vi "VS-Scale Time Axis.vi"(0 "Graph Ref":refnum<vi>, 7 "Running?":bool, 9 "Plot what":T1={"Mode"=enum."all time", "hours"=0.1} {"hours" min=0.1 max=24.0 step=0.5}, 11 "error in (no error)":errorcluster) -> (15 "error out":errorcluster)   [LabVIEW 2020]
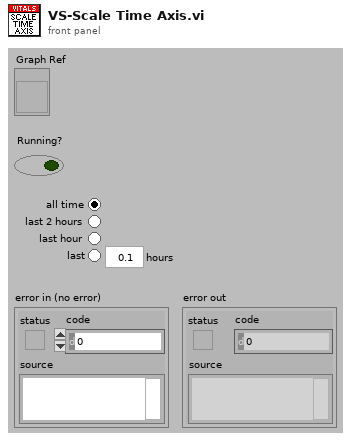
[diagram p1: front panel]
types:
  T1 = cluster{"Mode":enum32{"all time", "last 2 hours", "last hour", "last"}, "hours":dbl}
  T2 = enum32{"all time", "last 2 hours", "last hour", "last"}
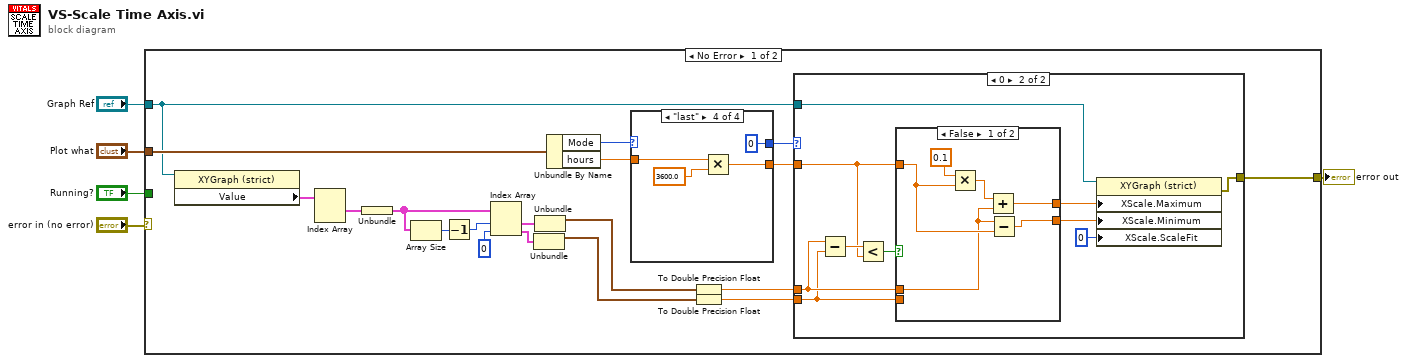
[diagram p0: block diagram]
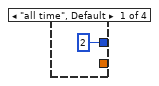
[diagram p2: hidden frame]
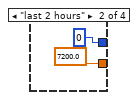
[diagram p3: hidden frame]
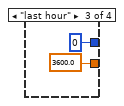
[diagram p4: hidden frame]
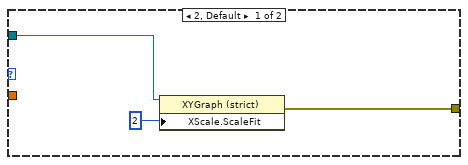
[diagram p5: hidden frame]
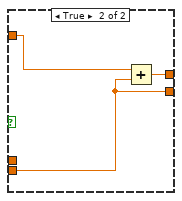
[diagram p6: hidden frame]
diagram:
  n1 = case shown="No Error" "error in (no error)" {
    selector: "error in (no error)" -> [_ w56]
    tunnel: [w23 w56] -> w4
    tunnel: "Plot what" -> [w24 _]
    tunnel: "Graph Ref" -> [w21 _]
    tunnel: "Running?" -> [_ _]
    frame No Error {
      n2 = property class="XYGraph (strict)"(reference=w21) -> ("Value"=w17:cluster{"Graph":cluster{timestamp, dbl}[]}[])  [unwired: 1 in, 2 out]
      n3 = Index Array(array=w17) -> (element #1=w19:cluster{"Graph":cluster{timestamp, dbl}[]})  [unwired: 2 in, 1 out]
      n4 = Unbundle(w19) -> ("Graph"=w20:cluster{timestamp, dbl}[])
      n5 = Array Size(array=w20) -> (size(s)=w18:i32)
      n6 = Decrement(x=w18) -> (x-1=w7:i32)
      n7 = Index Array(array=w20, index #1=w7, index #2=0 ("index")) -> (element #1=w15:cluster{timestamp, dbl}, element #2=w16:cluster{timestamp, dbl})
      n8 = Unbundle(w16) -> (w22:timestamp)  [unwired: 1 out]
      n9 = Unbundle(w15) -> (w10:timestamp)  [unwired: 1 out]
      n10 = Unbundle By Name(w24) -> ("Mode"=w14:T2, "hours"=w12:dbl)
      n11 = case shown="\"last\"" w14 {
        tunnel: [2 0 0 0] -> w11
        tunnel: [_ 7200.0 3600.0 w31] -> w13
        tunnel: w12 -> [_ _ _ w32]
        frame "all time", Default {
        }
        frame "last 2 hours" {
        }
        frame "last hour" {
        }
        frame "last" {
          n12 = Multiply(x=w32, y=3600.0) -> (x*y=w31:dbl)
        }
      }
      n13 = To Double Precision Float(number=w10) -> (double precision float=w9:dbl)
      n14 = To Double Precision Float(number=w22) -> (double precision float=w8:dbl)
      n15 = case shown="0" w11 {
        tunnel: w13 -> [_ w39]
        tunnel: w21 -> [w35 w43]
        tunnel: [w34 w42] -> w23
        tunnel: w9 -> [_ w41]
        tunnel: w8 -> [_ w37]
        frame 2, Default {
          n16 = property on="Property Node" class="XYGraph (strict)"(reference=w35, "XScale.ScaleFit"=u8 2 ("X Scale.Scale Fit")) -> (error out=w34:errorcluster)  [unwired: 1 in, 1 out]
        }
        frame 0 {
          n17 = Subtract(x=w41, y=w37) -> (x-y=w40:dbl)
          n18 = Less?(x=w40, y=w39) -> (x < y?=w38:bool)
          n19 = case shown="False" w38 {
            tunnel: [w52 w54] -> w45
            tunnel: [w51 w55] -> w44
            tunnel: w39 -> [w48 w53]
            tunnel: w41 -> [w47 _]
            tunnel: w37 -> [_ w54]
            frame False {
              n20 = Multiply(x=0.1, y=w48) -> (x*y=w49:dbl)
              n21 = Add(x=w49, y=w47) -> (x+y=w51:dbl)
              n22 = Subtract(x=w47, y=w48) -> (x-y=w52:dbl)
            }
            frame True {
              n23 = Add(x=w53, y=w54) -> (x+y=w55:dbl)
            }
          }
          n24 = property on="Property Node" class="XYGraph (strict)"(reference=w43, "XScale.Maximum"=w44, "XScale.Minimum"=w45, "XScale.ScaleFit"=u8 0 ("X Scale.Scale Fit")) -> (error out=w42:errorcluster)  [unwired: 1 in, 1 out]
        }
      }
    }
    frame Error {
    }
  }
  "error out" <- w4
